vi "Write Mode.vi"(8 "error in (no error)":errorcluster, 10 "Mode":enum16{"Running", "Shutdown"}(ring), 11 "Pound in":refnum<class "Pound.lvclass">) -> (0 "error out":errorcluster, 3 "Pound out":refnum<class "Pound.lvclass">)   [LabVIEW 2017, in "Pound.lvclass"]
uses:
  <vilib>/NI/Software Watchdog/Pound/Pound.lvclass
  <vilib>/NI/Software Watchdog/Pound/Pound.lvclass/Pound.ctl
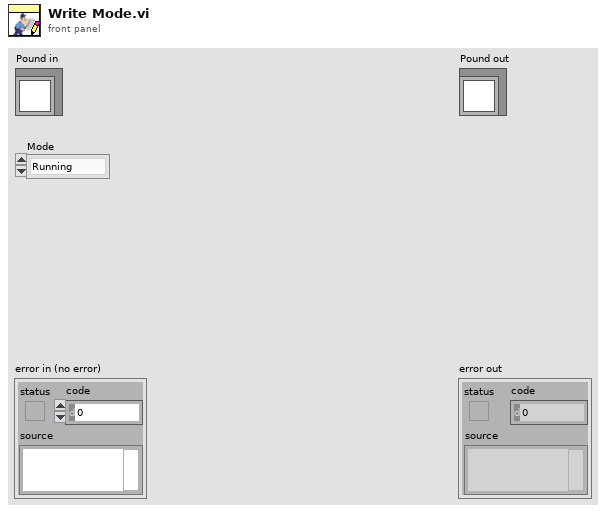
[diagram p1: front panel]
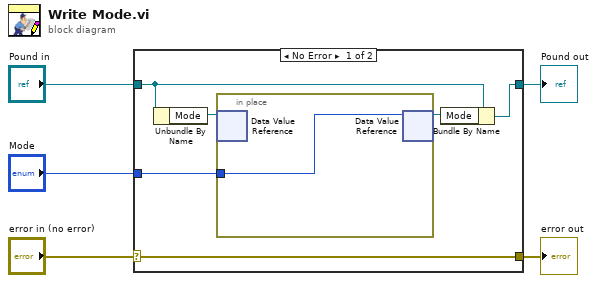
[diagram p0: block diagram]
diagram:
  n1 = case shown="No Error" "error in (no error)" {
    selector: "error in (no error)" -> [w11 w13]
    tunnel: [w11 w13] -> w4
    tunnel: [w10 w14] -> w2
    tunnel: "Pound in" -> [w9 w14]
    tunnel: "Mode" -> [w6 _]
    frame No Error {
      n2 = Unbundle By Name(w9) -> ("Mode"=w8:refnum<data-value>)
      n3 = in-place {
        in-place-border: w6 -> [w12]
        n4 = in-place-dvr #1(w8) -> ()  [unwired: 2 out]
        n5 = in-place-dvr #1(w12) -> (w7:refnum<data-value>)  [unwired: 1 out]
      }
      n6 = Bundle By Name(cluster=w9, "Mode"=w7) -> (w10:refnum<class "Pound.lvclass">)
    }
    frame Error {
    }
  }
  "error out" <- w4
  "Pound out" <- w2
